vi "Cream.vi"(8 "error in (no error)":errorcluster, 10 "Servo Pin":tag, 11 "Conv. Belt Pin":tag) -> (0 "error out 2":errorcluster)   [LabVIEW 2014]
uses:
  Controls/Conveyor Belt Functions.ctl
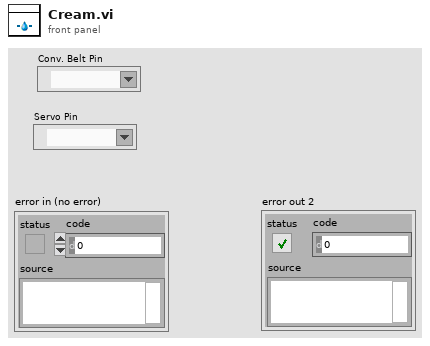
[diagram p1: front panel]
types:
  T1 = typedef "Conveyor Belt Functions.ctl" = enum16{"Move Forward", "Move Backward", "Stop"}
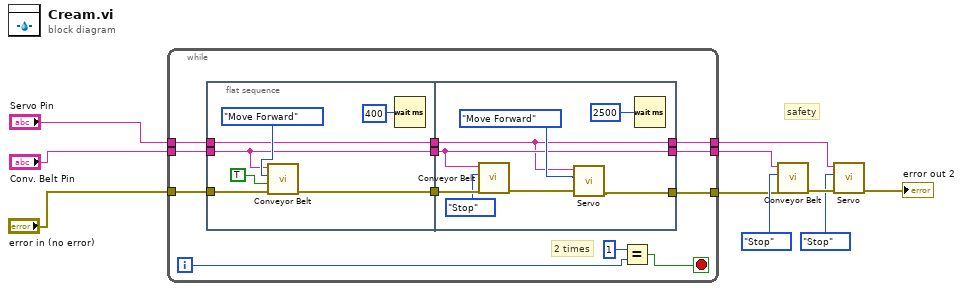
[diagram p0: block diagram]
diagram:
  # "safety"
  n1 = while {
    tunnel: "error in (no error)" -> [w22]
    tunnel: "Conv. Belt Pin" -> [w20]
    tunnel: [w19] -> w8
    tunnel: "Servo Pin" -> [w15]
    tunnel: [w12] -> w2
    tunnel: [w11] -> w1
    i -> [w17]
    stop <- w18 stop-if-true
    # "2 times"
    n2 = flat-sequence {
      tunnel: w22 -> [w29]
      tunnel: [w28] -> w21
      tunnel: w20 -> [w23]
      tunnel: w15 -> [w24]
      tunnel: [w24] -> w14
      tunnel: [w23] -> w13
      tunnel: w21 -> [w34]
      tunnel: [w36] -> w19
      tunnel: w14 -> [w30]
      tunnel: w13 -> [w31]
      tunnel: [w31] -> w12
      tunnel: [w30] -> w11
      frame #0 {
        n3 = call "Conveyor Belt.vi"("error in (no error)"=w29, "Slow"=TRUE, "Function"=Conveyor_Belt_Functions."Move Forward", "Conv. Belt Pin"=w23) -> ("error out"=w28:errorcluster)  [unwired: 7 in]
        n4 = Wait (ms)(milliseconds to wait=u32 400) -> ()  [unwired: 1 out]
      }
      frame #1 {
        n5 = call "Conveyor Belt.vi"("error in (no error)"=w34, "Function"=Conveyor_Belt_Functions."Stop", "Conv. Belt Pin"=w31) -> ("error out"=w33:errorcluster)  [unwired: 8 in]
        n6 = call "Servo.vi"("error in (no error)"=w33, "Function"=Conveyor_Belt_Functions."Move Forward", "Servo"=w30) -> ("error out"=w36:errorcluster)  [unwired: 8 in]
        n7 = Wait (ms)(milliseconds to wait=u32 2500) -> ()  [unwired: 1 out]
      }
    }
    n8 = Equal?(x=1, y=w17) -> (x = y?=w18:bool)
  }
  n9 = call "Conveyor Belt.vi"("error in (no error)"=w8, "Function"=Conveyor_Belt_Functions."Stop", "Conv. Belt Pin"=w2) -> ("error out"=w7:errorcluster)  [unwired: 8 in]
  n10 = call "Servo.vi"("error in (no error)"=w7, "Function"=Conveyor_Belt_Functions."Stop", "Servo"=w1) -> ("error out"=→"error out 2":errorcluster)  [unwired: 8 in]
